vi "Select DAQmx Channels.vi"(2 "Channels Out":string[](array[string]), 8 "error in (no error)":errorcluster, 9 "Sensor List":refnum<class "Sensor List Class.lvclass">) -> (0 "error out":errorcluster)   [LabVIEW 2013]
uses:
  lib/Data Access Objects/Metadata/Persistant DAO Actions.ctl
  lib/Data Access Objects/Sensors/Sensor List Class.lvclass
panel:
  in  "Done":bool
  in  "Select Channels":i32[](listbox)
  in  "Tasks":u16(ring) caption="OM  Location"
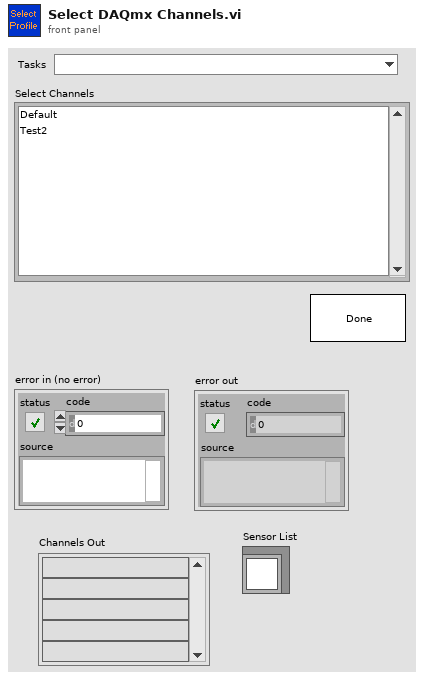
[diagram p1: front panel]
types:
  T1 = typedef "Persistant DAO Actions.ctl" = enum16{"Init", "Get", "Set", "Load", "Save"}
  T2 = typedef "DAQMx Tasks.ctl" = cluster{"LBCB1 Readings":refnum<k21>, "LBCB2 Readings":refnum<k21>, "LBCB1 Commands":refnum<k21>, "LBCB2 Commands":refnum<k21>, "Sensors":refnum<k21>[]}
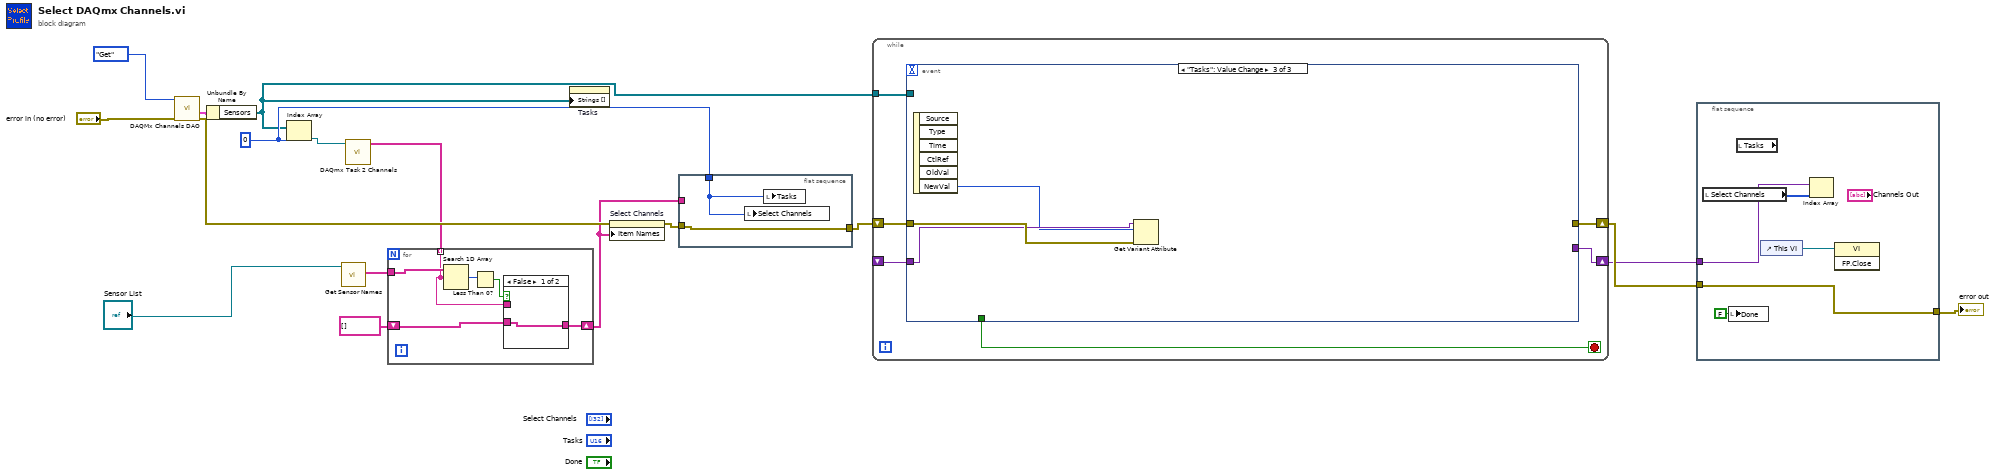
[diagram p0: block diagram]
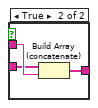
[diagram p2: hidden frame]
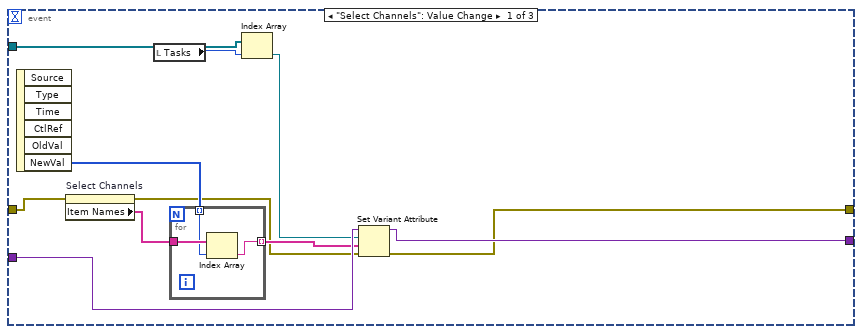
[diagram p3: hidden frame]
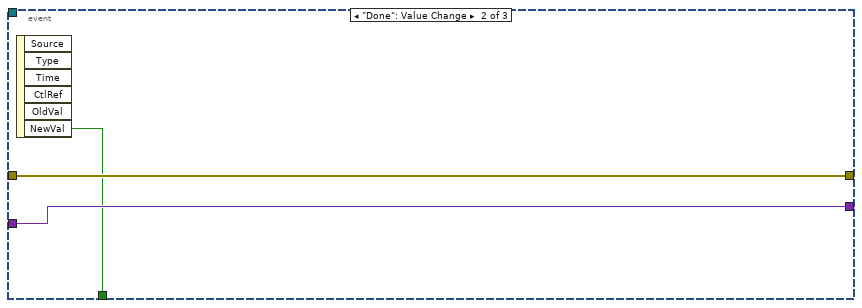
[diagram p4: hidden frame]
diagram:
  w3 = 0 ("index")
  n1 = call "DAQMx Channels DAO.vi"("error in (no error)"="error in (no error)", "Actions"=Persistant_DAO_Actions."Get") -> ("error out"=w9:errorcluster, "Names Out"=w10:T2)  [unwired: 7 in, 1 out]
  n2 = Unbundle By Name(w10) -> ("Sensors"=w1:refnum<k21>[])
  n3 = Index Array(array=w1, index=w3) -> (element=w8:refnum<k21>)
  n4 = call "Get Sensor Names.vi"("Sensor List Class in"="Sensor List") -> ("Names"=w5:string[])  [unwired: 8 in, 2 out]
  n5 = call "DAQmx Task 2 Channels.vi"("DAQmx Task Name"=w8) -> ("Channels Out"=w6:string[])  [unwired: 10 in]
  n6 = for {
    tunnel: w6 -> [w20] mode=indexing
    tunnel: w5 -> [w23]
    shift-right: [w19] -> w2
    shift-left: string[] [] -> [w18]
    n7 = Search 1D Array(1D array=w23, element=w20) -> (index of element=w22:i32)  [unwired: 1 in]
    n8 = Less Than 0?(x=w22) -> (x < 0?=w21:bool)
    n9 = case shown="False" w21 {
      tunnel: w20 -> [_ w27]
      tunnel: [w24 w26] -> w19
      tunnel: w18 -> [w24 w25]
      frame False {
      }
      frame True {
        n10 = Build Array (concatenate)(w25, w27) -> (w26:string[])
      }
    }
  }
  n11 = property on="Tasks" class="Ring (strict)"("Strings []"=w1) -> ()  [unwired: 2 in, 2 out]
  n12 = property on="Select Channels" class="LstBox (strict)"(error in=w9, "Item Names"=w2) -> (error out=w17:errorcluster)  [unwired: 1 in, 1 out]
  n13 = flat-sequence {
    tunnel: w2 -> [_]
    tunnel: w17 -> [w29]
    tunnel: [w29] -> w13
    tunnel: w3 -> [w28]
    frame #0 {
      n14 = local write "Select Channels"(w28) -> ()
      n15 = local write "Tasks"(w28) -> ()
    }
  }
  n16 = while {
    shift-right: [w33] -> w16
    shift-left: w13 -> [w34]
    shift-right: [w32] -> w14
    shift-left: _ -> [w35]
    tunnel: w1 -> [w30]
    stop <- w31 stop-if-true
    n17 = event shown="[2] \"Tasks\": Value Change" {
      selector: _ -> [_ _ _]
      dyn-events: _ -> [_ _ _]
      timeout: _ -> [_ _ _]
      tunnel: w35 -> [w44 w52 w54]
      tunnel: w34 -> [w41 w51 w55]
      tunnel: [w36 w51 w56] -> w33
      tunnel: [w43 w52 _] -> w32
      tunnel: [_ w50 _] -> w31
      tunnel: w30 -> [w46 _ _]
      event "Select Channels": Value Change {
        n18 = event-data() -> ("NewVal"=w39:i32[])  [unwired: 1 in, 5 out]
        n19 = property on="Select Channels" class="LstBox (strict)"(error in=w41) -> (error out=w37:errorcluster, "Item Names"=w40:string[])  [unwired: 1 in, 1 out]
        n20 = local read "Tasks"() -> (w45:u16)
        n21 = for {
          tunnel: w40 -> [w49]
          tunnel: w39 -> [w48] mode=indexing
          tunnel: [w47] -> w38 mode=indexing
          n22 = Index Array(array=w49, index=w48) -> (element=w47:string)
        }
        n23 = Index Array(array=w46, index=w45) -> (element=w42:refnum<k21>)
        n24 = Set Variant Attribute(Variant=w44, name=w42, value=w38, error in=w37) -> (Variant out=w43:variant, error out=w36:errorcluster)  [unwired: 1 out]
      }
      event "Done": Value Change {
        n25 = event-data() -> ("NewVal"=w50:bool)  [unwired: 1 in, 5 out]
      }
      event "Tasks": Value Change {
        n26 = event-data() -> ("NewVal"=w53:u16)  [unwired: 1 in, 5 out]
        n27 = Get Variant Attribute(Variant=w54, name=w53, error in=w55) -> ()  [unwired: 1 in, 4 out]
      }
    }
  }
  n28 = flat-sequence {
    tunnel: w16 -> [w60]
    tunnel: [w60] -> w15
    tunnel: w14 -> [w59]
    frame #0 {
      n29 = local read "Select Channels"() -> (w58:i32[])
      n30 = local write "Done"(FALSE ("Ok")) -> ()
      n31 = local read "Tasks"() -> ()  [unwired: 1 out]
      n32 = control-ref of="This VI"() -> (w57:refnum<vi>)
      n33 = Index Array(array=w59, index=w58) -> ()  [unwired: 1 out]
      n34 = invoke class="VI" method="FP.Close"(reference=w57) -> ()  [unwired: 2 in, 3 out]
    }
  }
  "error out" <- w15
